vi "LHF.DB.MongoDB.vi"() -> ()   [LabVIEW 2013]
uses:
  src/LHF.DB.Mongo.lvclass
panel:
  out "Pass":bool
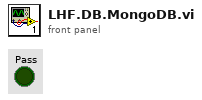
[diagram p1: front panel]
types:
  T1 = cluster{"name":string, "data":dbl[][], "newAttribute":string}
  T2 = cluster{"JSON Update":string, "JSON Update":string}
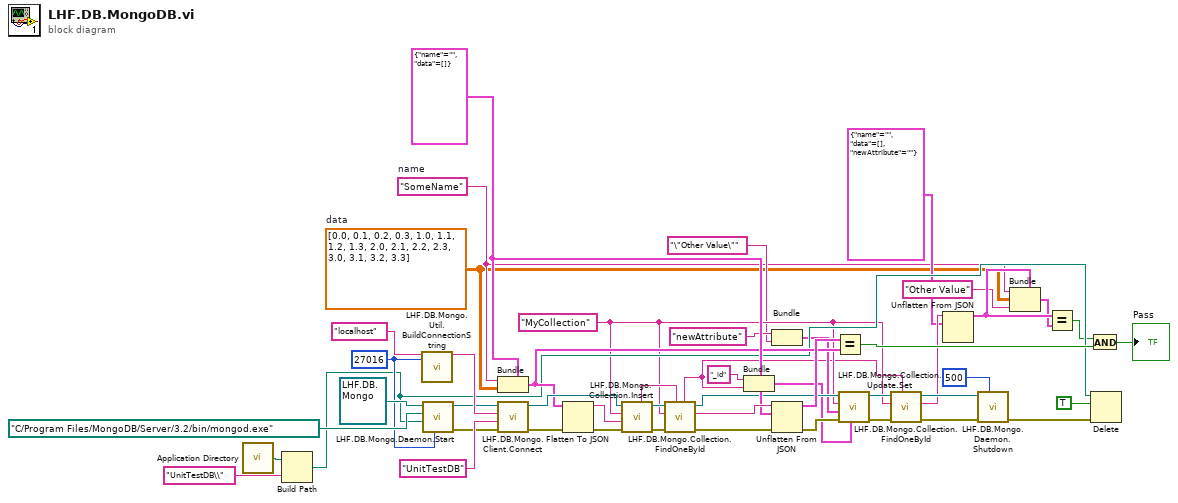
[diagram p0: block diagram]
diagram:
  w6 = "SomeName"  # name
  w5 = dbl[][] [[0.0, 0.1, 0.2, 0.3], [1.0, 1.1, 1.2, 1.3], [2.0, 2.1, 2.2, 2.3], [3.0, 3.1, 3.2, 3.3]]  # data
  w33 = cluster{"name":string, "data":dbl[][]} {"name"="", "data"=[]}
  w16 = "MyCollection" ("Collection")
  w46 = u32 27016 ("Port (27017)")
  n1 = call <vilib>:"Application Directory.vi"() -> ("Application Directory"=w25:path)
  n2 = Build Path(base path=w25, name or relative path="UnitTestDB\\") -> (appended path=w23:path)
  n3 = call "LHF.DB.Mongo.Util.BuildConnectionString.vi"("host"="localhost", "port"=w46) -> ("connectionString"=w45:string)  [unwired: 17 in]
  n4 = call-dynamic "LHF.DB.Mongo.Daemon.Start.vi"("Port (27017)"=w46, "data folder"=w23, "mongod path"=path "C:/Program Files/MongoDB/Server/3.2/bin/mongod.exe", "LHF.DB.Mongo in"=refnum<class "LHF.DB.Mongo.lvclass"> refnum) -> ("error out"=w42:errorcluster, "LHF.DB.Mongo out"=w43:refnum<class "LHF.DB.Mongo.lvclass">)  [unwired: 6 in]
  n5 = Bundle(cluster=w33, "name"=w6, "data"=w5) -> (w29:cluster{"name":string, "data":dbl[][]})
  n6 = call-dynamic "LHF.DB.Mongo.Client.Connect.vi"("error in (no error)"=w42, "database"="UnitTestDB", "url"=w45, "LHF.DB.Mongo in"=w43) -> ("error out"=w32:errorcluster, "LHF.DB.Mongo out"=w40:refnum<class "LHF.DB.Mongo.lvclass">)  [unwired: 6 in]
  n7 = Flatten To JSON(anything=w29, error in (no error)=w32) -> (JSON string=w39:string, 11:w31:errorcluster)  [unwired: 1 in]
  n8 = call-dynamic "LHF.DB.Mongo.Collection.Insert.vi"("error in (no error)"=w31, "JSON Document"=w39, "Collection"=w16, "LHF.DB.Mongo"=w40) -> ("error out"=w37:errorcluster, "LHF.DB.Mongo out"=w38:refnum<class "LHF.DB.Mongo.lvclass">, "ObjectID out"=w36:string)  [unwired: 4 in, 1 out]
  n9 = call-dynamic "LHF.DB.Mongo.Collection.FindOneById.vi"("ObjectID in"=w36, "error in (no error)"=w37, "Collection"=w16, "LHF.DB.Mongo in"=w38) -> ("error out"=w34:errorcluster, "Document"=w35:string, "LHF.DB.Mongo out"=w22:refnum<class "LHF.DB.Mongo.lvclass">, "ObjectID"=w10:string)  [unwired: 4 in]
  n10 = Bundle("JSON Update"="_id", "ObjectID"=w10) -> (w14:cluster{"JSON Update":string, "ObjectID":string})  [unwired: 1 in]
  n11 = Bundle("JSON Update"="newAttribute", "JSON Update"="\"Other Value\"") -> (w11:T2)  [unwired: 1 in]
  n12 = Unflatten From JSON(JSON string=w35, type and defaults=w33, error in (no error)=w34) -> (value=w30:cluster{"name":string, "data":dbl[][]}, error out=w21:errorcluster)  [unwired: 4 in]
  n13 = Equal?(x=w30, y=w29) -> (x = y?=w28:bool)
  n14 = call-dynamic "LHF.DB.Mongo.Collection.Update.Set.vi"("Query"=w14, "error in (no error)"=w21, "Update"=w11, "Collection"=w16, "LHF.DB.Mongo in"=w22) -> ("error out"=w18:errorcluster, "LHF.DB.Mongo out"=w20:refnum<class "LHF.DB.Mongo.lvclass">)  [unwired: 5 in]
  n15 = call-dynamic "LHF.DB.Mongo.Collection.FindOneById.vi"("ObjectID in"=w10, "error in (no error)"=w18, "Collection"=w16, "LHF.DB.Mongo in"=w20) -> ("error out"=w17:errorcluster, "Document"=w9:string, "LHF.DB.Mongo out"=w19:refnum<class "LHF.DB.Mongo.lvclass">)  [unwired: 4 in, 1 out]
  n16 = Unflatten From JSON(JSON string=w9, type and defaults=T1 {"name"="", "data"=[], "newAttribute"=""}) -> (value=w7:T1)  [unwired: 5 in, 1 out]
  n17 = call-dynamic "LHF.DB.Mongo.Daemon.Shutdown.vi"("timeout"=500, "error in (no error)"=w17, "LHF.DB.Mongo in"=w19) -> ("error out"=w27:errorcluster)  [unwired: 7 in, 1 out]
  n18 = Bundle(cluster=w7, "name"=w6, "data"=w5, "newAttribute"="Other Value") -> (w3:T1)
  n19 = Equal?(x=w7, y=w3) -> (x = y?=w1:bool)
  n20 = And(x=w1, y=w28) -> (x .and. y?=→"Pass":bool)
  n21 = Delete(path (use dialog)=w23, entire hierarchy (F)=TRUE, error in=w27) -> ()  [unwired: 2 in, 3 out]
